vi "SetState_SelectedItem.vi"(8 "error in (no error)":errorcluster caption="错误输入（无错误）", 10 "选中记录":string, 11 "TCPServerClass输入":refnum<class "TCPServerClass.lvclass">) -> (0 "error out":errorcluster caption="错误输出", 3 "TCPServerClass输出":refnum<class "TCPServerClass.lvclass">)   [LabVIEW 2019, in "TCPServerClass.lvclass"]
uses:
  TCPServerClass.lvclass
  TCPServerClass.lvclass/TCPServerClass.ctl
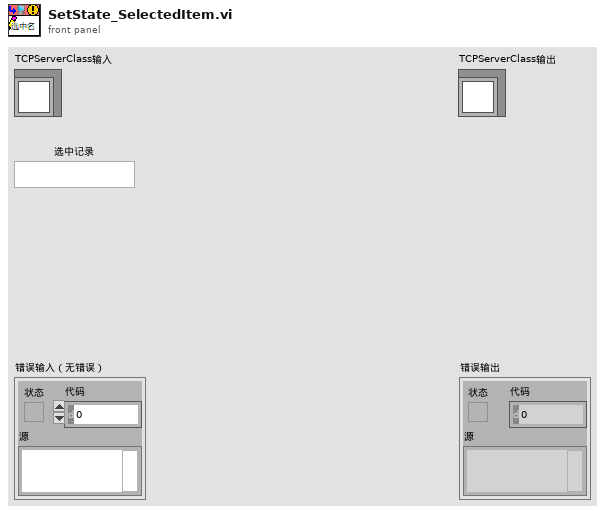
[diagram p1: front panel]
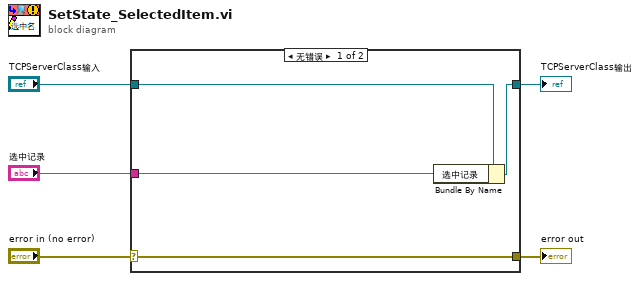
[diagram p0: block diagram]
diagram:
  n1 = case shown="无错误" "error in (no error)" {
    selector: "error in (no error)" -> [w9 w10]
    tunnel: [w9 w10] -> w4
    tunnel: [w7 w11] -> w2
    tunnel: "TCPServerClass输入" -> [w8 w11]
    tunnel: "选中记录" -> [w6 _]
    frame No Error {
      n2 = Bundle By Name(cluster=w8, "选中记录"=w6) -> (w7:refnum<class "TCPServerClass.lvclass">)
    }
    frame Error {
    }
  }
  "error out" <- w4
  "TCPServerClass输出" <- w2
